vi "Asynchronous - Update BC to RT Data - Preprocess Map.vi"(8 "error in (no error)":errorcluster, 11 "Map (BC to RT)":T2[](array[typedef]) {"Channel Data Reference" format="%.0x"}) -> (0 "error out":errorcluster, 3 "Frames":T1[](array[typedef]))   [LabVIEW 2017, in "Ballard MIL-1553 Engine.lvlib"]
uses:
  Ballard MIL-1553 Engine.lvlib
  Controls/RT Async_Map BC2RT.ctl
  <vilib>/NI Veristand/Custom Device API/Data Reference.ctl
  Controls/RT Async_Map_Type.ctl
  Controls/Asynchronous - Update BC to RT Data - Map.ctl
  <vilib>/NI VeriStand/Custom Device Tools/Custom Device Utility Library/Custom Device Utility Library.lvlib
  <vilib>/NI VeriStand/Custom Device API/Custom Device API.lvlib
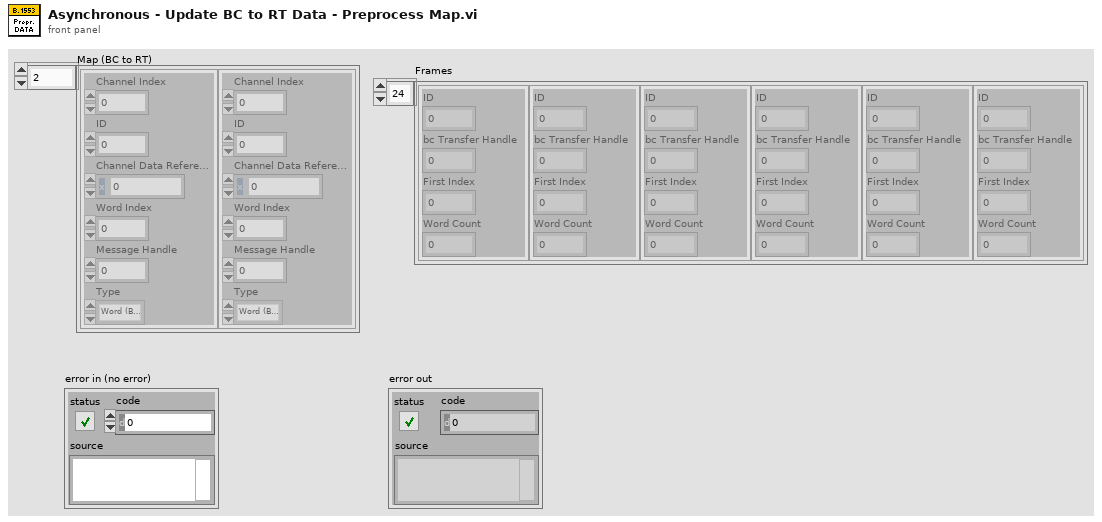
[diagram p1: front panel]
types:
  T1 = typedef "Ballard MIL-1553 Engine.lvlib/Asynchronous - Update BC to RT Data - Map.ctl" = cluster{"ID":i32, "bc Transfer Handle":u64, "First Index":i32, "Word Count":i32}
  T2 = typedef "Ballard MIL-1553 Engine.lvlib/RT Async_Map BC2RT.ctl" = cluster{"Channel Index":i32, "ID":i32, "Channel Data Reference":T3, "Word Index":i32, "Message Handle":u64, "Type":T4}
  T3 = typedef "Custom Device API.lvlib/Data Reference.ctl" = i32
  T4 = typedef "Ballard MIL-1553 Engine.lvlib/RT Async_Map_Type.ctl" = enum16{"Word (BC to RT)", "Word (MC (Rx))", "Acyclic Message Trigger", "Word (RT to ..)", "Word (RT to RT)", "Word (MC (Tx))", "RT Status", "BC Commands", "RT Commands"}
  T5 = cluster{"ID":i32, "bc Transfer Handle":u64, "Indexes":i32[]}[]
  T6 = cluster{"ID":i32, "bc Transfer Handle":u64, "Indexes":i32[]}
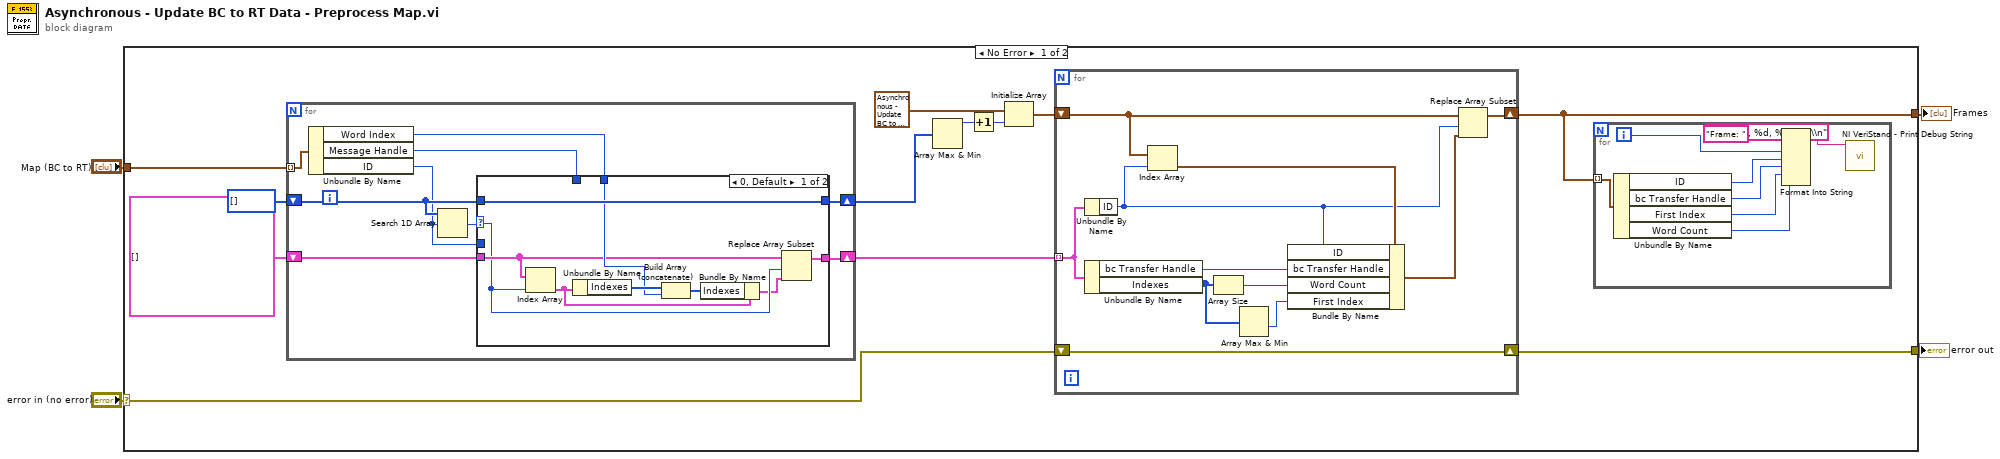
[diagram p0: block diagram]
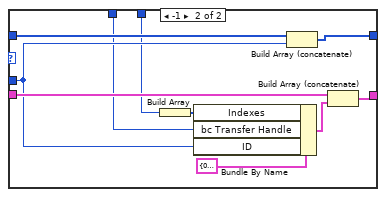
[diagram p2: hidden frame]
diagram:
  n1 = case shown="No Error" "error in (no error)" {
    selector: "error in (no error)" -> [w11 w65]
    tunnel: [w10 w65] -> w3
    tunnel: "Map (BC to RT)" -> [w16 _]
    tunnel: [w5 _] -> w1
    frame No Error {
      n2 = for {
        tunnel: w16 -> [w45] mode=indexing
        shift-right: [w38] -> w7
        shift-left: i32[] [] -> [w42]
        shift-right: [w37] -> w6
        shift-left: T5 [] -> [w43]
        n3 = Unbundle By Name(w45) -> ("Word Index"=w39:i32, "Message Handle"=w40:u64, "ID"=w41:i32)
        n4 = Search 1D Array(1D array=w42, element=w41) -> (index of element=w44:i32)  [unwired: 1 in]
        n5 = case shown="0, Default" w44 {
          selector: w44 -> [w50 _]
          tunnel: w43 -> [w51 w61]
          tunnel: w42 -> [w54 w64]
          tunnel: w41 -> [_ w58]
          tunnel: w40 -> [_ w57]
          tunnel: w39 -> [w52 w56]
          tunnel: [w54 w63] -> w38
          tunnel: [w46 w59] -> w37
          frame 0, Default {
            n6 = Index Array(array=w51, index=w50) -> (element=w49:T6)
            n7 = Unbundle By Name(w49) -> ("Indexes"=w53:i32[])
            n8 = Build Array (concatenate)(w53, w52) -> (w48:i32[])
            n9 = Bundle By Name(cluster=w49, "Indexes"=w48) -> (w47:T6)
            n10 = Replace Array Subset(array=w51, new element=w47, index=w50) -> (w46:T5)
          }
          frame -1 {
            n11 = Build Array(w56) -> (w55:i32[])
            n12 = Bundle By Name(cluster=T6 {"ID"=0, "bc Transfer Handle"=0, "Indexes"=[]}, "Indexes"=w55, "bc Transfer Handle"=w57, "ID"=w58) -> (w60:T6)
            n13 = Build Array (concatenate)(w64, w58) -> (w63:i32[])
            n14 = Build Array (concatenate)(w61, w60) -> (w59:T5)
          }
        }
      }
      n15 = Array Max & Min(array=w7) -> (max value=w15:i32)  [unwired: 3 out]
      n16 = Increment(x=w15) -> (x+1=w14:i32)
      n17 = Initialize Array(T1 {"ID"=-1, "bc Transfer Handle"=18446744073709551615, "First Index"=-1, "Word Count"=-1} ("Map Entry"), w14) -> (w12:T1[])
      n18 = for {
        shift-right: [w34] -> w5
        shift-left: w12 -> [w35]
        shift-right: [w36] -> w10
        shift-left: w11 -> [w36]
        tunnel: w6 -> [w30] mode=indexing
        n19 = Unbundle By Name(w30) -> ("ID"=w31:i32)
        n20 = Unbundle By Name(w30) -> ("bc Transfer Handle"=w29:u64, "Indexes"=w27:i32[])
        n21 = Index Array(array=w35, index=w31) -> (element=w33:T1)
        n22 = Array Size(array=w27) -> (size(s)=w28:i32)
        n23 = Array Max & Min(array=w27) -> (min value=w26:i32)  [unwired: 3 out]
        n24 = Bundle By Name(cluster=w33, "ID"=w31, "bc Transfer Handle"=w29, "Word Count"=w28, "First Index"=w26) -> (w32:T1)
        n25 = Replace Array Subset(array=w35, new element=w32, index=w31) -> (w34:T1[])
      }
      n26 = for {
        tunnel: w5 -> [w25] mode=indexing
        i -> [w23]
        n27 = Unbundle By Name(w25) -> ("ID"=w22:i32, "bc Transfer Handle"=w21:u64, "First Index"=w20:i32, "Word Count"=w19:i32)
        n28 = Format Into String(format string="%d, %d, %d, %d, %d\\n", initial string="Frame: ", w23, w22, w21, w20, w19) -> (resulting string=w18:string)  [unwired: 1 in, 1 out]
        n29 = call <vilib>:"NI VeriStand - Print Debug String.vi"("Message"=w18) -> ()  [unwired: 10 in, 1 out]
      }
    }
    frame Error {
    }
  }
  "error out" <- w3
  "Frames" <- w1
